vi "Generate GUID.vi"(8 "error in (no error)":errorcluster) -> (0 "error out":errorcluster, 3 "GUID":string)   [LabVIEW 2018, in "Instrument Addon Scripting API.lvlib"]
uses:
  Instrument Addon Scripting API.lvlib
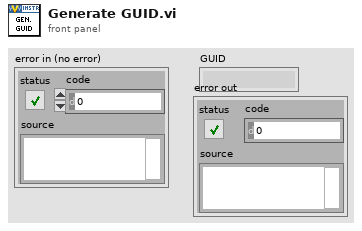
[diagram p1: front panel]
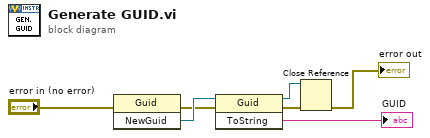
[diagram p0: block diagram]
diagram:
  n1 = invoke class="Guid" method="NewGuid"(error in="error in (no error)") -> (error out=w3:errorcluster, "NewGuid"=w4:refnum<k24>)  [unwired: 2 in, 1 out]
  n2 = invoke class="Guid" method="ToString"(reference=w4, error in=w3) -> (reference out=w5:refnum<k24>, error out=w2:errorcluster, "ToString"=→"GUID":string)  [unwired: 1 in]
  n3 = Close Reference(reference=w5, error in (no error)=w2) -> (error out=→"error out":errorcluster)
